vi "Execute Publication Policy.vi"(7 "Default PublicationPolicy":refnum<class "IPublicationPolicy.lvclass">, 9 "Last Publish Time":timestamp, 10 "Last Published Value":variant, 11 "MutexedPublishRequest":refnum<class "MutexedPublishRequest.lvclass">) -> (0 "error out (Reject Publication)":errorcluster, 1 "Publication Time":timestamp, 2 "Value to Publish":variant)   [LabVIEW 2017, in "IMediator.lvlib" / "MutexedPublishRequest.lvclass"]
doc: "This method decides whether or not to send or otherwise handle the new data value. The policy is set and maintained by the subscriber. The Topic Actor knows no policy details, it just passes the new value in. If there is a failure inside this method, the Topic Actor must assume the listener is no longer valid (dead/unrecoverable) and should delete it from the Subscriber list.\n\n<License>\nCopyright © 2017 Composed Systems, LLC | All rights reserved\nwww.composed.io\n\nAuthor: Ethan Stern <ethan.stern@composed.io>\n\nThis software is provided \"AS IS\" WITHOUT WARRANTIES, either express or implied, AND IS FOR EDUCATIONAL PURPOSES ONLY.\n</License>"
uses:
  MutexedPublishRequest.lvclass
  C:/Git/mva-framework/Source/Framework/IMediator/PublishRequest/PublishRequest.lvclass
  IPublicationPolicy/IPublicationPolicy.lvclass
  PublishRequest/PublishRequest.lvclass/PublishRequest.ctl
  MutexedPublishRequest.lvclass/MutexedPublishRequest.ctl
  gpm_packages/@cs/transport/Source/ITransport/ITransport.lvclass
  PublishRequest/PublishRequest.lvclass
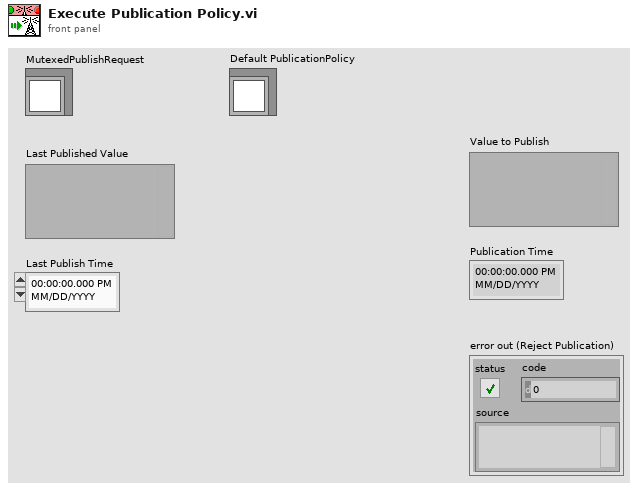
[diagram p1: front panel]
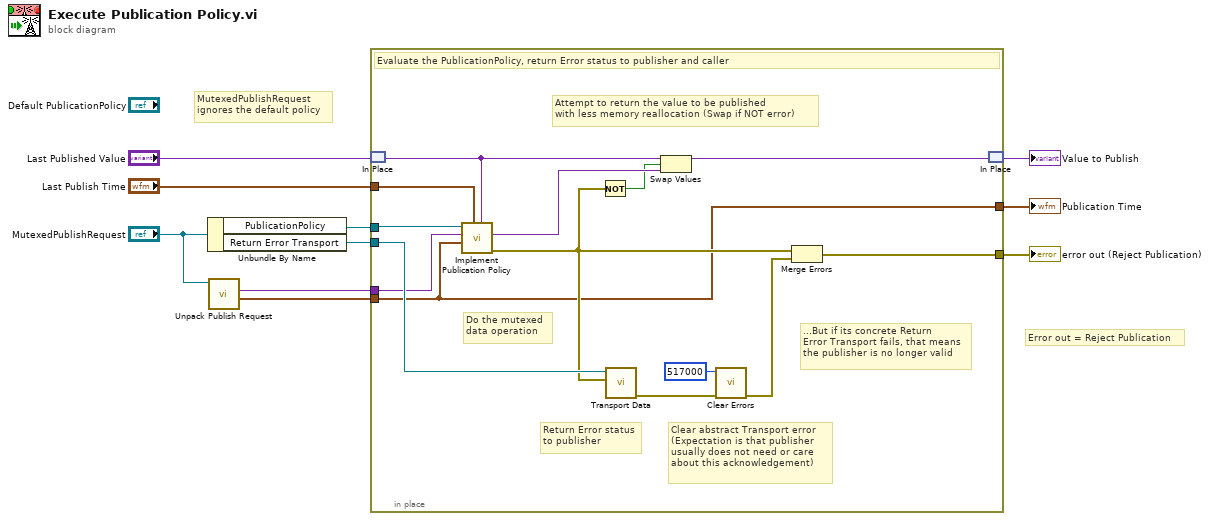
[diagram p0: block diagram]
diagram:
  # "MutexedPublishRequest\nignores the default policy"
  # "Error out = Reject Publication"
  n1 = Unbundle By Name("MutexedPublishRequest") -> ("PublicationPolicy"=w6:refnum<class "IPublicationPolicy.lvclass">, "Return Error Transport"=w7:refnum<class "ITransport.lvclass">)
  n2 = call "Unpack Publish Request.vi"("PublishRequest In"="MutexedPublishRequest") -> ("Publication Time"=w4:timestamp, "Value"=w5:variant)  [unwired: 7 in, 2 out]
  n3 = in-place {
    in-place-border: [w20] -> w10
    in-place-border: w7 -> [w19]
    in-place-border: w6 -> [w15]
    in-place-border: w5 -> [w14]
    in-place-border: w4 -> [w11]
    in-place-border: "Last Publish Time" -> [w12]
    in-place-border: [w11] -> w1
    # "Do the mutexed\ndata operation"
    # "Attempt to return the value to be published\nwith less memory reallocation (Swap if NOT error)"
    # "...But if its concrete Return\nError Transport fails, that means\nthe publisher is no longer valid"
    # "Return Error status\nto publisher"
    # "Clear abstract Transport error\n(Expectation is that publisher\nusually does not need or care\nabout this acknowledgement)"
    # "Evaluate the PublicationPolicy, return Error status to publisher and caller"
    n4 = in-place-match #1("Last Published Value") -> (w13:variant)
    n5 = call-dynamic "Implement Publication Policy.vi"("Last Published Value"=w13, "Last Published Time"=w12, "New Value Time"=w11, "New Value"=w14, "PublicationPolicy"=w15) -> ("error out (Reject Publication)"=w17:errorcluster, "Value to Publish"=w18:variant)  [unwired: 5 in]
    n6 = Not(x=w17) -> (.not. x?=w16:bool)
    n7 = call "Transport Data.vi"("Value"=w17, "ITransport in"=w19) -> ("error out"=w24:errorcluster)  [unwired: 8 in, 1 out]
    n8 = Swap Values(12:w13, 13:w16, 14:w18) -> (1:w21:variant)  [unwired: 1 out]
    n9 = call <vilib>:"Clear Errors.vi"("error in (no error)"=w24, "specific error code to clear (0: all)"=517000) -> ("error out"=w23:errorcluster)  [unwired: 4 in, 1 out]
    n10 = Merge Errors(w17, w23) -> (w20:errorcluster)
    n11 = in-place-match #1(w21) -> (→"Value to Publish":variant)
  }
  "error out (Reject Publication)" <- w10
  "Publication Time" <- w1
